vi "Create New Data.vi"() -> (2 "New Value":refnum<user-event>, 3 "Data out":refnum<class "Data.lvclass">)   [LabVIEW 2017, in "Filled Text Fields.lvlib" / "Data.lvclass"]
uses:
  Data.lvclass
  Data.PrivateData.ctl
  Data.lvclass/Data.ctl
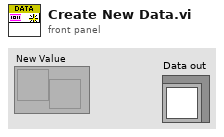
[diagram p1: front panel]
types:
  T1 = typedef "Filled Text Fields.lvlib/Data.lvclass/Data.PrivateData.ctl" = cluster{"Data":string}
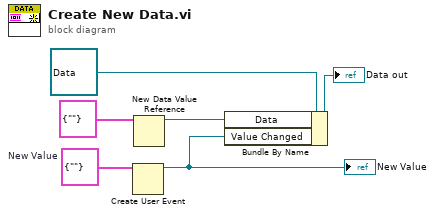
[diagram p0: block diagram]
diagram:
  w2 = T1 {"Data"=""}  # New Value
  n1 = Create User Event(user event datatype=w2) -> (user event=w1:refnum<user-event>)  [unwired: 1 in, 1 out]
  "New Value" <- w1
  n2 = New Data Value Reference(data value=T1 {"Data"=""} ("Data")) -> (data value reference=w3:refnum<data-value>)  [unwired: 1 in, 1 out]
  n3 = Bundle By Name(cluster=refnum<class "Data.lvclass"> refnum ("Data in"), "Data"=w3, "Value Changed"=w1) -> (→"Data out":refnum<class "Data.lvclass">)
